vi "Receive Message.vi"(6 "priority":i32, 10 "Actor in in":refnum<class "Actor.lvclass">, 11 "Message in":refnum<class "Message.lvclass">) -> (0 "error out":errorcluster, 2 "Actor out":refnum<class "Actor.lvclass">)   [LabVIEW 2013, in "Actor Framework.lvlib" / "Actor.lvclass"]
doc: "This VI should be overriden ONLY if you are creating a proxy actor for remote transmission. If you are, override this VI to transmit the received message to a new destination, maintaining the given priority."
uses:
  <vilib>/ActorFramework/Actor/Actor.lvclass
  <vilib>/ActorFramework/Message/Message.lvclass
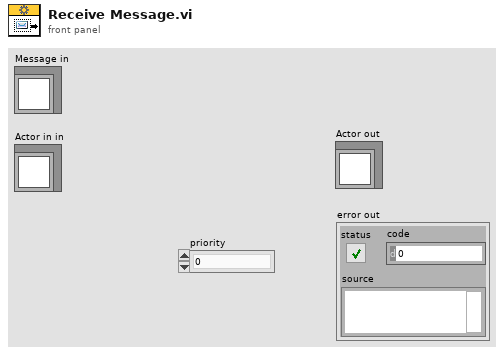
[diagram p1: front panel]
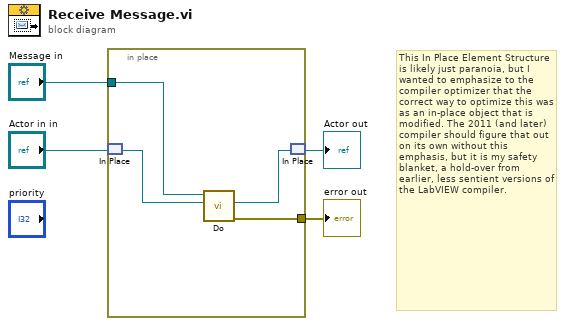
[diagram p0: block diagram]
diagram:
  # "This In Place Element Structure is likely just paranoia, but I wanted to emphasize to the compiler optimizer that the correct way to optimize this was as an in-place object that is modified. The 2011 (and later) compiler should figure that out on its own without this emphasis, but it is my safety blanket, a hold-over from earlier, less sentient versions of the LabVIEW compiler."
  n1 = in-place {
    in-place-border: [w8] -> w4
    in-place-border: "Message in" -> [w7]
    n2 = in-place-match #1("Actor in in") -> (w6:refnum<class "Actor.lvclass">)
    n3 = call-dynamic "Do.vi"("Actor in"=w6, "Message"=w7) -> ("error out"=w8:errorcluster, "Actor out"=w5:refnum<class "Actor.lvclass">)  [unwired: 8 in]
    n4 = in-place-match #1(w5) -> (→"Actor out":refnum<class "Actor.lvclass">)
  }
  "error out" <- w4
